vi "Basic Tester.vi"() -> ()   [LabVIEW 2023, in "Error Manager.lvlib" / "Testers.lvlib"]
uses:
  Testers.lvlib
  Error Manager.lvlib
  Pop-up New Error Dialogue Setting (enum).ctl
  <vilib>/Utility/sysdir.llb/System Directory Type.ctl
panel:
  out "error out":errorcluster
  in  "Error code":i32=-1
  in  "Show call chain?":bool=TRUE
  in  "Error message":string="Dummy error (testing)"
  in  "Error?":bool
  in  "Stop Tester":bool
  out "EHL iteration":i32
  in  "Generate Error":bool
  # "Basic Tester\n\nInstructions\n1. Run the VI\n2. Press 'Generate Error' to generate an error.\n    - If you wish, you can change the Error code, the Error Message, and whether the call chain is to be contained in the error message or not.\n3. Press the 'No error/Error' button to bring up the Error Manager GUI (in other words, to show the Front Panel of the Error Handler asynchronous module). This is analogous to how a user would press bring up the Error Manager GUI in a real application that uses the Error Handler.\n4. Inspect the Error Manager GUI. Use the buttons/controls/indicators available in the Error Manager GUI.\n    - Navigate to or open the Error Log text file"
  # "This button simulates the 'No error/Error' button placed somewhere in the main GUI of the calling app (for example, on the top or bottom bars of the calling app). You can copy-paste this button into the GUI of the calling app if you wish."
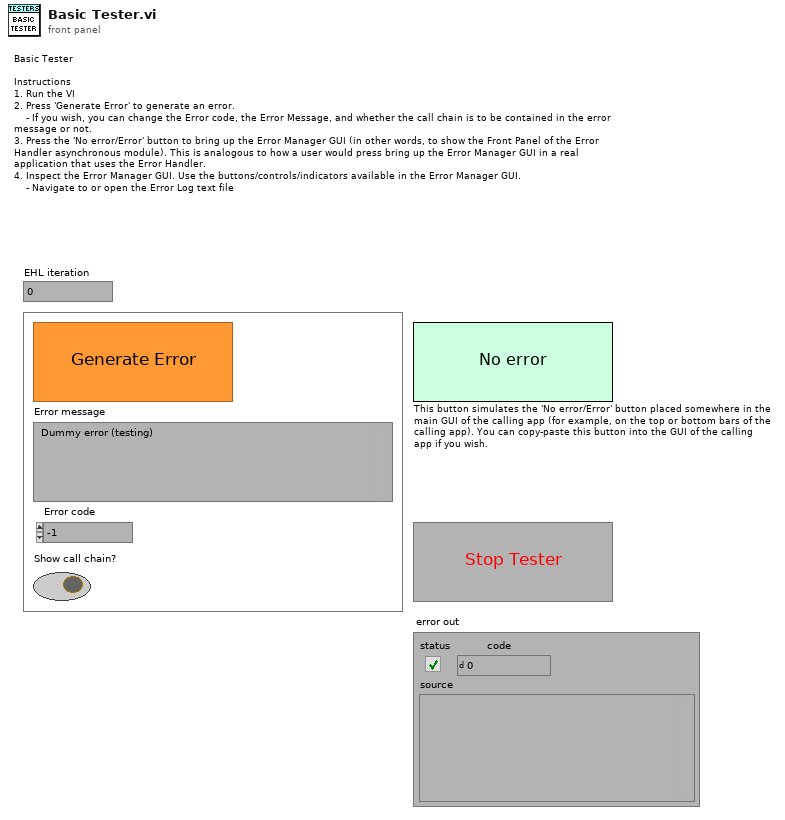
[diagram p1: front panel]
types:
  T1 = typedef "Error Manager.lvlib/Pop-up New Error Dialogue Setting (enum).ctl" = enum16{"Pop-up New Error Dialogue", "Don't pop-up New Error Dialogue"}
  T2 = typedef "System Directory Type.ctl" = i32
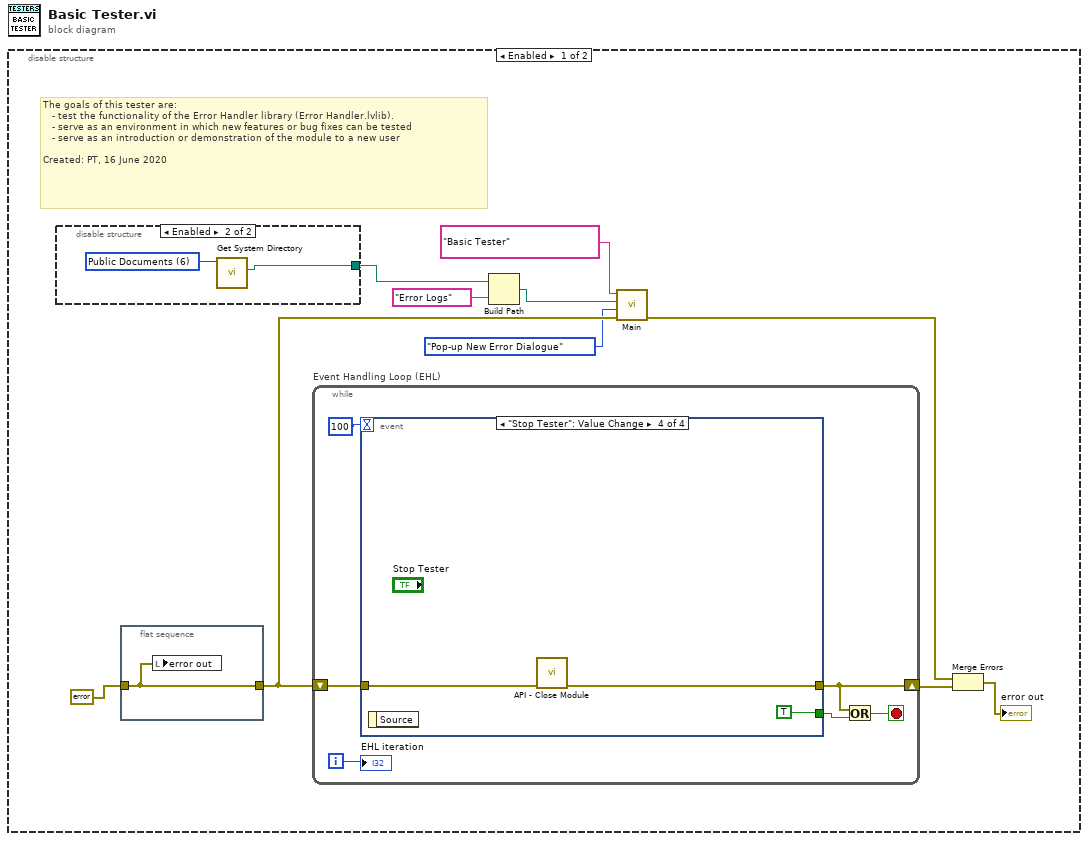
[diagram p0: block diagram]
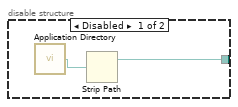
[diagram p2: hidden frame]
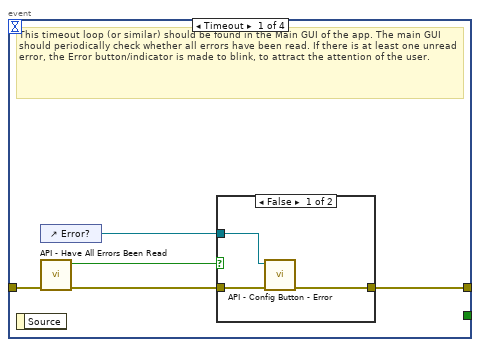
[diagram p3: hidden frame]
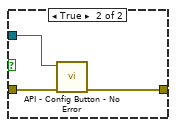
[diagram p4: hidden frame]
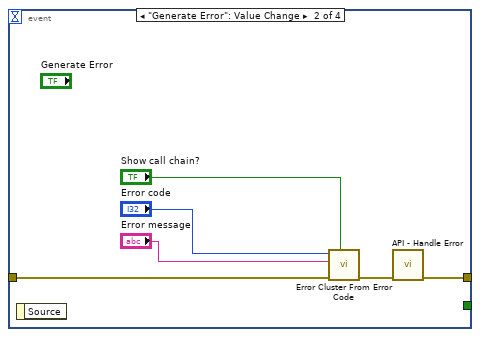
[diagram p5: hidden frame]
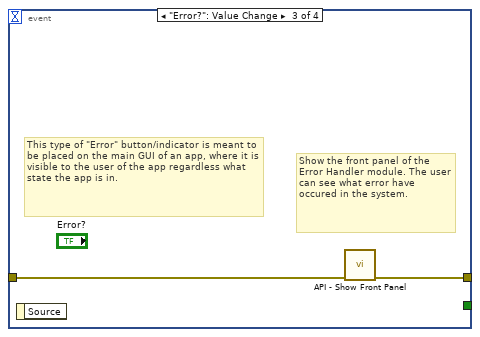
[diagram p6: hidden frame]
diagram:
  n1 = disable-structure shown="Enabled" {
    frame Enabled {
      # "The goals of this tester are:\n   - test the functionality of the Error Handler library (Error Handler.lvlib).\n   - serve as an environment in which new features or bug fixes can be tested\n   - serve as an introduction or demonstration of the module to a new user\n\nCreated: PT, 16 June 2020"
      n2 = disable-structure shown="Enabled" {
        disable-tunnel: [w11 w13] -> w4
        frame Disabled {
          n3 = call <vilib>:"Application Directory.vi"() -> ("Application Directory"=w12:path)
          n4 = Strip Path(path=w12) -> (stripped path=w11:path)  [unwired: 1 out]
        }
        frame Enabled {
          w14 = T2 6 items=["User Home"=0, "User Desktop"=1, "User Documents"=2, "User Application Data"=3, "User Preferences"=4, "User Temporary"=5, "Public Documents"=6, "Public Application Data"=7, "Public Preferences"=8, "Public Cache"=13, "System Core Libraries"=9, "System Installed Libraries"=10, "Application Files"=11, "Boot Volume Root"=12] ("system directory type")
          n5 = call <vilib>:"Get System Directory.vi"("system directory type"=w14) -> ("system directory"=w13:path)  [unwired: 10 in]
        }
      }
      n6 = flat-sequence {
        tunnel: [w15] -> w7
        tunnel: errorcluster {"status"=FALSE, "code"=0, "source"=""} ("error constant") -> [w15]
        frame #0 {
          n7 = local write "error out"(w15) -> ()
        }
      }
      n8 = while "Event Handling Loop (EHL)" {
        shift-right: [w18] -> w9
        shift-left: w7 -> [w19]
        i -> [w21]
        stop <- w16 stop-if-true
        n9 = event shown="[3] \"Stop Tester\": Value Change" {
          selector: _ -> [_ _ _ _]
          dyn-events: _ -> [_ _ _ _]
          timeout: 100 -> [_ _ _ _]
          tunnel: w19 -> [w26 w36 w40 w42]
          tunnel: [w24 w38 w39 w43] -> w18
          tunnel: [_ _ _ TRUE] -> w17
          event Timeout {
            # "This timeout loop (or similar) should be found in the Main GUI of the app. The main GUI should periodically check whether all errors have been read. If there is at least one unread error, the Error button/indicator is made to blink, to attract the attention of the user."
            n10 = event-data() -> ()  [unwired: 1 in, 1 out]
            n11 = control-ref of="Error?"() -> (w22:refnum<vi>)
            n12 = call "API - Have All Errors Been Read.vi"("error in"=w26) -> ("error out"=w25:errorcluster, "Have All Errors Been Read?"=w23:bool)  [unwired: 9 in]
            n13 = case shown="False" w23 {
              tunnel: [w27 w31] -> w24
              tunnel: w25 -> [w28 w32]
              tunnel: w22 -> [w29 w30]
              frame False {
                n14 = call "API - Config Button - Error.vi"("error in"=w28, "Error Button"=w29) -> ("error out"=w27:errorcluster)  [unwired: 9 in]
              }
              frame True {
                n15 = call "API - Config Button - No Error.vi"("error in"=w32, "Error Button"=w30) -> ("error out"=w31:errorcluster)  [unwired: 9 in]
              }
            }
          }
          event "Generate Error": Value Change {
            n16 = event-data() -> ()  [unwired: 1 in, 1 out]
            n17 = call <vilib>:"Error Cluster From Error Code.vi"("show call chain? (False)"="Show call chain?", "error in (no error)"=w36, "error message (\"\")"="Error message", "error code (0)"="Error code") -> ("error out"=w37:errorcluster)  [unwired: 5 in]
            n18 = call "API - Handle Error.vi"("error in"=w37) -> ("error out"=w38:errorcluster)  [unwired: 10 in]
          }
          event "Error?": Value Change {
            # "This type of \"Error\" button/indicator is meant to be placed on the main GUI of an app, where it is visible to the user of the app regardless what state the app is in."
            # "Show the front panel of the Error Handler module. The user can see what error have occured in the system."
            n19 = event-data() -> ()  [unwired: 1 in, 1 out]
            n20 = call "API - Show Front Panel.vi"("error in"=w40) -> ("error out"=w39:errorcluster)  [unwired: 10 in]
          }
          event "Stop Tester": Value Change {
            n21 = event-data() -> ()  [unwired: 1 in, 1 out]
            n22 = call "API - Close Module.vi"("error in"=w42) -> ("error out"=w43:errorcluster)  [unwired: 10 in]
          }
        }
        n23 = Or(x=w18, y=w17) -> (x .or. y?=w16:bool)
        "EHL iteration" <- w21
      }
      n24 = Build Path(base path=w4, name or relative path="Error Logs") -> (appended path=w2:path)
      n25 = call "Main.vi"("Error In"=w7, "Pop-up New Error Dialogue Setting (Default = Pop-up Dialogue)"=Pop-up_New_Error_Dialogue_Setting_(enum)."Pop-up New Error Dialogue", "The folder to store the Error Logs"=w2, "Test Rig Name or Acronym"="Basic Tester" ("Jig Name or Acronym")) -> ("Error Out"=w10:errorcluster)  [unwired: 7 in]
      n26 = Merge Errors(w10, w9) -> (→"error out":errorcluster)
    }
    frame Disabled {
    }
  }
